vi "总磷单步调试对话框.vi"() -> ()   [LabVIEW 2016, in "斯坦道总氮.lvlib"]
panel:
  in  "停止":bool
  out "注射器温度":sgl
  out "消解温度":sgl
  out "ADC":sgl
  out "F3":sgl format="%#.6f"
  out "F2":sgl format="%#.6f"
  out "F1":sgl format="%#.6f"
  out "F0":sgl format="%#.6f"
  in  "退出":bool
  in  "启动":bool
  in  "总磷氨氮调试":u16[](xcontrol)
  # "单步调试界面"
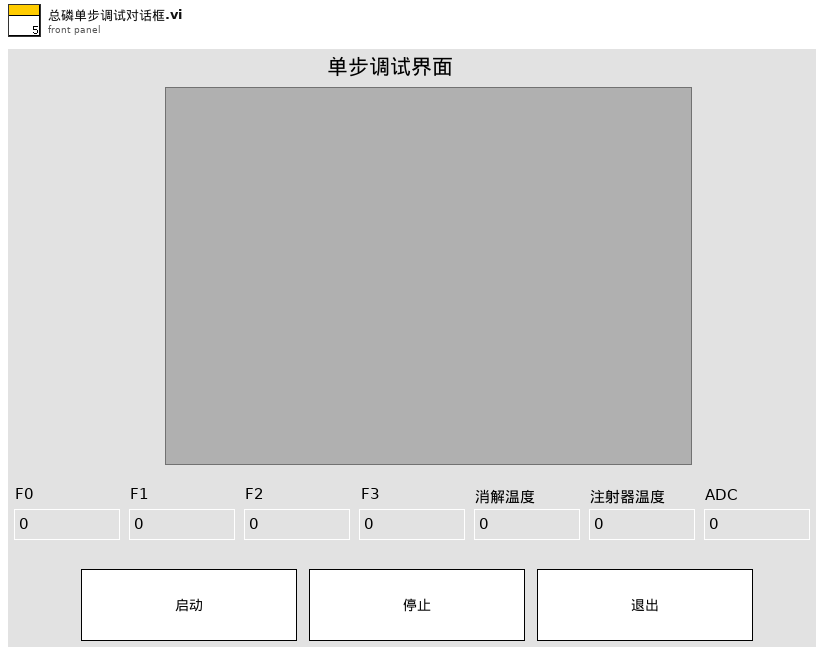
[diagram p1: front panel]
types:
  T1 = typedef "调试控件V3.xctl/仪器类型.ctl" = enum16{"A版", "B版"}
  T2 = cluster{"系统时间":timestamp, "工作状态":u16, "测量模式":enum16{"待机", "连续模式", "周期模式", "定点模式", "受控模式", "手动模式"}, "告警代码":u16, "故障代码":u16, "日志代码":u16, "软件版本":u16, "F0":sgl, "F1":sgl, "F2":sgl, "F3":sgl, "T":sgl, "H":sgl, "id":u16, "flowid":u16, "量程":u16, "总磷控温温度1":sgl, "营养盐控温温度2":sgl, "ADC":sgl}
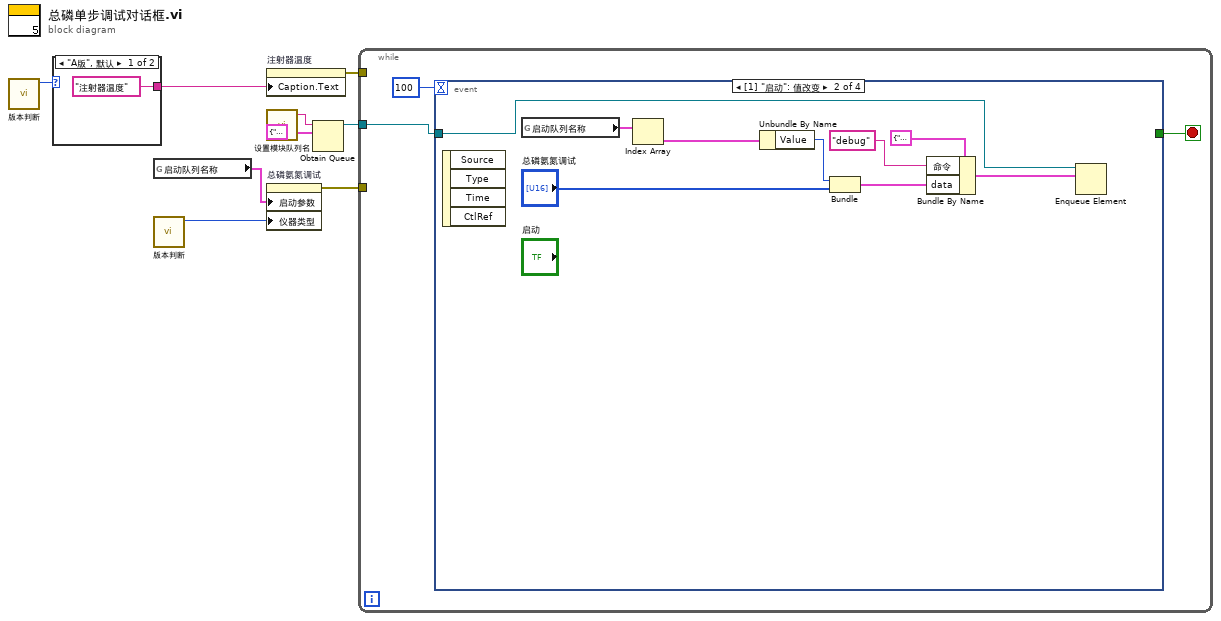
[diagram p0: block diagram]
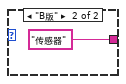
[diagram p2: hidden frame]
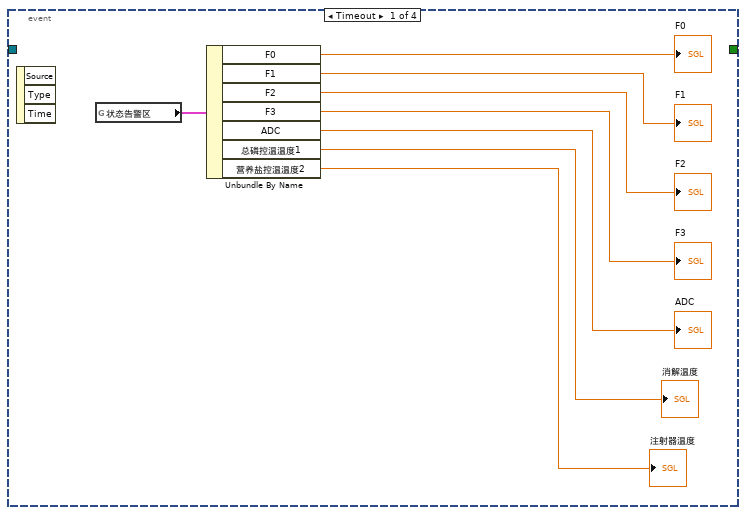
[diagram p3: hidden frame]
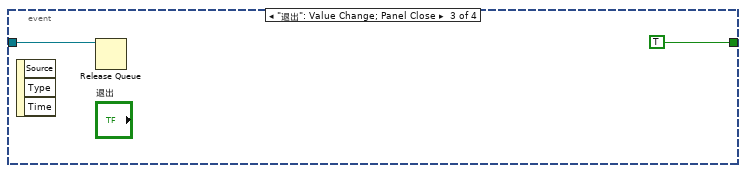
[diagram p4: hidden frame]
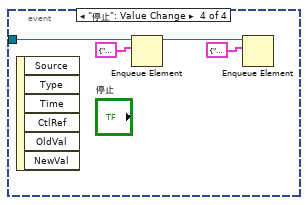
[diagram p5: hidden frame]
diagram:
  n1 = call "版本判断.vi"() -> ("仪器类型"=w3:T1)  [unwired: 11 in]
  n2 = case shown="\"A版\", 默认" w3 {
    tunnel: ["注射器温度" ("标题.文本") "传感器" ("标题.文本")] -> w2
    frame "A版", Default {
    }
    frame "B版" {
    }
  }
  n3 = global read "model config var.vi" "启动队列名称"() -> (w5:cluster{"String":string, "Value":u16}[])
  n4 = call "版本判断.vi"() -> ("仪器类型"=w4:T1)  [unwired: 11 in]
  n5 = property on="注射器温度" class="DigNum (严格)"("Caption.Text"=w2) -> (error out=w1:errorcluster)  [unwired: 2 in, 1 out]
  n6 = call "设置模块队列名.vi"() -> ("Msg"=w6:string)  [unwired: 5 in]
  n7 = property on="总磷氨氮调试" class="调试控件V3 (严格)"("启动参数"=w5, "仪器类型"=w4) -> (error out=w7:errorcluster)  [unwired: 2 in, 1 out]
  n8 = Obtain Queue(name (unnamed)=w6, element data type=cluster{"命令":string, "data":variant} {"命令"="", "data"=variant}) -> (queue out=w8:refnum<queue>)  [unwired: 3 in, 2 out]
  n9 = while {
    tunnel: w8 -> [w14]
    tunnel: w7 -> [_]
    tunnel: w1 -> [_]
    stop <- w13 stop-if-true
    n10 = event shown="[1] \"启动\": 值改变" {
      selector: _ -> [_ _ _ _]
      dyn-events: _ -> [_ _ _ _]
      timeout: 100 -> [_ _ _ _]
      tunnel: w14 -> [_ w27 w32 w34]
      tunnel: [_ _ TRUE _] -> w13
      event Timeout {
        n11 = event-data() -> ()  [unwired: 1 in, 3 out]
        n12 = global read "VAR总磷总氮全局变量.vi" "状态告警区"() -> (w15:T2)
        n13 = Unbundle By Name(w15) -> ("F0"=→"F0":sgl, "F1"=→"F1":sgl, "F2"=→"F2":sgl, "F3"=→"F3":sgl, "ADC"=→"ADC":sgl, "总磷控温温度1"=→"消解温度":sgl, "营养盐控温温度2"=→"注射器温度":sgl)
      }
      event "启动": Value Change {
        n14 = event-data() -> ()  [unwired: 1 in, 4 out]
        n15 = global read "model config var.vi" "启动队列名称"() -> (w23:cluster{"String":string, "Value":u16}[])
        n16 = Index Array(array=w23) -> (element=w25:cluster{"String":string, "Value":u16})  [unwired: 1 in]
        n17 = Unbundle By Name(w25) -> ("Value"=w24:u16)
        n18 = Bundle("Value"=w24, "总磷氨氮调试"="总磷氨氮调试") -> (w28:cluster{"Value":u16, "总磷氨氮调试":u16[]})  [unwired: 1 in]
        n19 = Bundle By Name(cluster=cluster{"命令":string, "data":variant} {"命令"="", "data"=variant} ("元素"), "命令"="debug", "data"=w28) -> (w29:cluster{"命令":string, "data":variant})
        n20 = Enqueue Element(queue=w27, element=w29) -> ()  [unwired: 2 in, 3 out]
      }
      event "退出": Value Change; Panel Close {
        n21 = event-data() -> ()  [unwired: 1 in, 3 out]
        n22 = Release Queue(queue=w32) -> ()  [unwired: 2 in, 3 out]
      }
      event "停止": Value Change {
        n23 = event-data() -> ()  [unwired: 1 in, 6 out]
        n24 = Enqueue Element(queue=w34, element=cluster{"命令":string, "data":variant} {"命令"="启动", "data"=variant(cluster{"站号":u16, "控制命令输出":u16[]} {"站号"=1, "控制命令输出"=[2816]})} ("元素")) -> (queue out=w35:refnum<queue>)  [unwired: 2 in, 2 out]
        n25 = Enqueue Element(queue=w35, element=cluster{"命令":string, "data":variant} {"命令"="启动", "data"=variant(cluster{"站号":u16, "控制命令输出":u16[]} {"站号"=2, "控制命令输出"=[2816]})} ("元素")) -> ()  [unwired: 2 in, 3 out]
      }
    }
  }
